vi "Change User Access Level.vi"(6 "Array of Permissions":bool[](array[boolean]), 8 "error in (no error)":errorcluster, 9 "Access":T1=enum."Guest", 10 "Username":string, 11 "UserPwd DB in":refnum<class "UserPwd DB.lvclass">) -> (0 "error out":errorcluster, 2 "changed":bool, 3 "UserPwd DB out":refnum<class "UserPwd DB.lvclass">)   [LabVIEW 2016, in "UserPwd DB.lvlib" / "UserPwd DB.lvclass"]
uses:
  <userlib>/Common Components/UserPwd DB/UserPwd DB/UserPwd DB.lvclass
  <userlib>/Common Components/UserPwd DB/UserPwd DB/Access Level.ctl
  <userlib>/Common Components/UserPwd DB/UserPwd DB/UserPwd DB.lvclass/UserPwd DB.ctl
  <userlib>/Common Components/UserPwd DB/UserPwd DB/Data saved.ctl
  <vilib>/Utility/error.llb/Error Cluster From Error Code.vi
  <vilib>/ErrorRing/Error Ring.xnode
  <vilib>/addons/_JKI.lib/Serialization/JSON/JKI JSON Serialization.lvlib
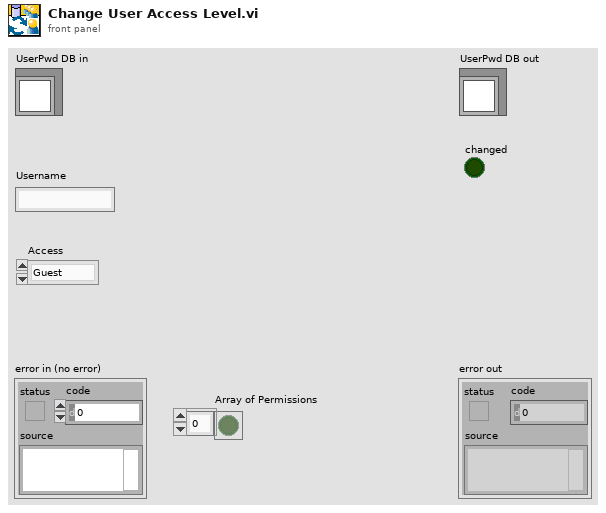
[diagram p1: front panel]
types:
  T1 = typedef "UserPwd DB.lvlib/UserPwd DB.lvclass/Access Level.ctl" = enum16{"Admin", "User lv1", "User lv2", "User lv3", "User lv4", "User lv5", "User lv6", "User lv7", "User lv8", "User lv9", "Guest"}
  T2 = typedef "UserPwd DB.lvlib/UserPwd DB.lvclass/Data saved.ctl" = cluster{"Encrypted Password":string, "Access":T1, "Permission":u32}
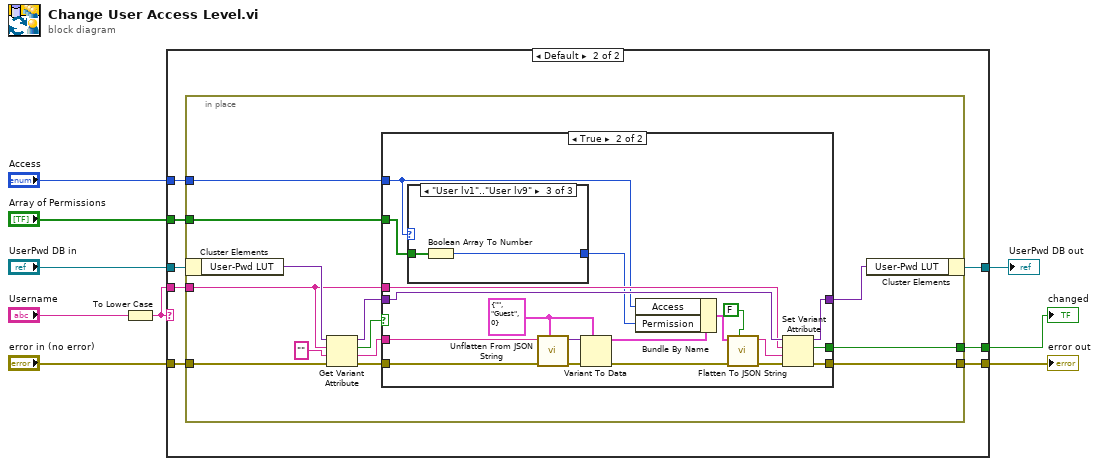
[diagram p0: block diagram]
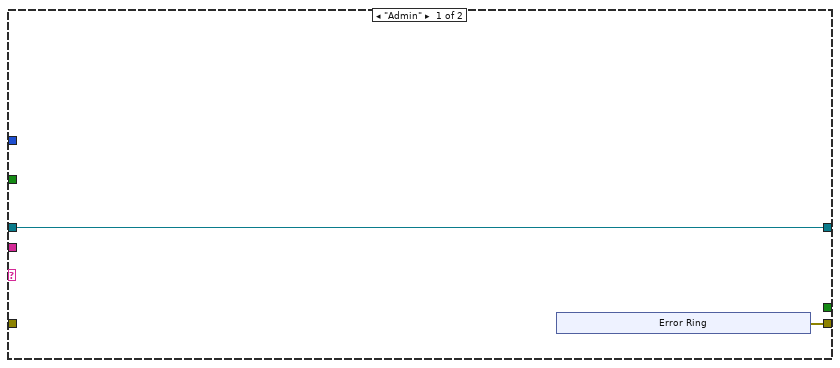
[diagram p2: hidden frame]
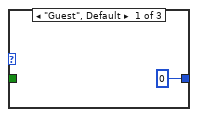
[diagram p4: hidden frame]
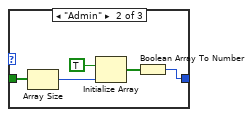
[diagram p5: hidden frame]
diagram:
  n1 = To Lower Case(string="Username") -> (all lower case string=w2:string)
  n2 = case shown="Default" w2 {
    tunnel: "UserPwd DB in" -> [w11 w23]
    tunnel: [w11 w22] -> w8
    tunnel: w2 -> [_ w21]
    tunnel: "error in (no error)" -> [_ w20]
    tunnel: [w10 w19] -> w6
    tunnel: [_ w18] -> w5
    tunnel: "Access" -> [_ w17]
    tunnel: "Array of Permissions" -> [_ w16]
    frame "Admin" {
      n3 = xnode "Error Ring"() -> ("error out"=w10:errorcluster)
    }
    frame Default {
      n4 = in-place {
        in-place-border: w21 -> [w32]
        in-place-border: w20 -> [w34]
        in-place-border: [w27] -> w19
        in-place-border: [w29] -> w18
        in-place-border: w17 -> [w30]
        in-place-border: w16 -> [w24]
        n5 = in-place-cluster #1(w23) -> ("User-Pwd LUT"=w36:variant)
        n6 = Get Variant Attribute(Variant=w36, name=w32, default value (empty Variant)="" ("Password"), error in=w34) -> (duplicate Variant=w35:variant, found=w26:bool, value=w31:string, error out=w28:errorcluster)
        n7 = case shown="True" w26 {
          tunnel: w35 -> [w38 w57]
          tunnel: [w38 w56] -> w33
          tunnel: w32 -> [_ w55]
          tunnel: w31 -> [_ w50]
          tunnel: w30 -> [_ w42]
          tunnel: [_ w54] -> w29
          tunnel: w28 -> [w37 w53]
          tunnel: [w37 w52] -> w27
          tunnel: w24 -> [_ w41]
          frame False {
          }
          frame True {
            w47 = T2 {"Encrypted Password"="", "Access"=enum."Guest", "Permission"=0} ("Data")
            n8 = case shown="\"User lv1\"..\"User lv9\"" w42 {
              tunnel: w41 -> [_ w63 w65]
              tunnel: [u32 0 w59 w64] -> w40
              frame "Guest", Default {
              }
              frame "Admin" {
                n9 = Array Size(array=w63) -> (size(s)=w61:i32)
                n10 = Initialize Array(TRUE, w61) -> (w60:bool[])
                n11 = Boolean Array To Number(Boolean array=w60) -> (number=w59:u32)
              }
              frame "User lv1".."User lv9" {
                n12 = Boolean Array To Number(Boolean array=w65) -> (number=w64:u32)
              }
            }
            n13 = call <vilib>:"Unflatten From JSON String.vi"("Type and Defaults"=w47, "error in (no error)"=w53, "JSON String"=w50) -> ("error out"=w51:errorcluster, "Variant"=w48:variant)  [unwired: 7 in]
            n14 = Variant To Data(error in=w51, type=w47, Variant=w48) -> (data=w46:T2, error out=w49:errorcluster)
            n15 = Bundle By Name(cluster=w46, "Access"=w42, "Permission"=w40) -> (w44:T2)
            n16 = call <vilib>:"Flatten To JSON String.vi"("Multiline (T)"=FALSE, "error in (no error)"=w49, "Variant"=w44) -> ("error out"=w45:errorcluster, "JSON String"=w43:string)  [unwired: 7 in]
            n17 = Set Variant Attribute(Variant=w57, name=w55, value=w43, error in=w45) -> (Variant out=w56:variant, replaced=w54:bool, error out=w52:errorcluster)
          }
        }
        n18 = in-place-cluster #1("User-Pwd LUT"=w33) -> (w22:refnum<class "UserPwd DB.lvclass">)
      }
    }
  }
  "error out" <- w6
  "UserPwd DB out" <- w8
  "changed" <- w5
